vi "AuMT8852B EDR Carrier Frequency and Modulation Extended Results.vi"(5 "Stage":T1(ring), 8 "error in (no error)":errorcluster, 11 "VISA session":refnum<visa-resource-name>) -> (0 "error out":errorcluster, 2 "error code":i32, 3 "VISA session out":refnum<visa-resource-name>, 4 "Results":T2)   [LabVIEW 2017]
doc: "Anritsu MT8852B Bluetooth Tester\n\nReturns the results of the EDR Carrier Frequency Stability and Modulation test.\n\nINPUTS\nStage - results of the individual hopping stages of the test.\n\nOUTPUTS\nResults - measurements made during the test."
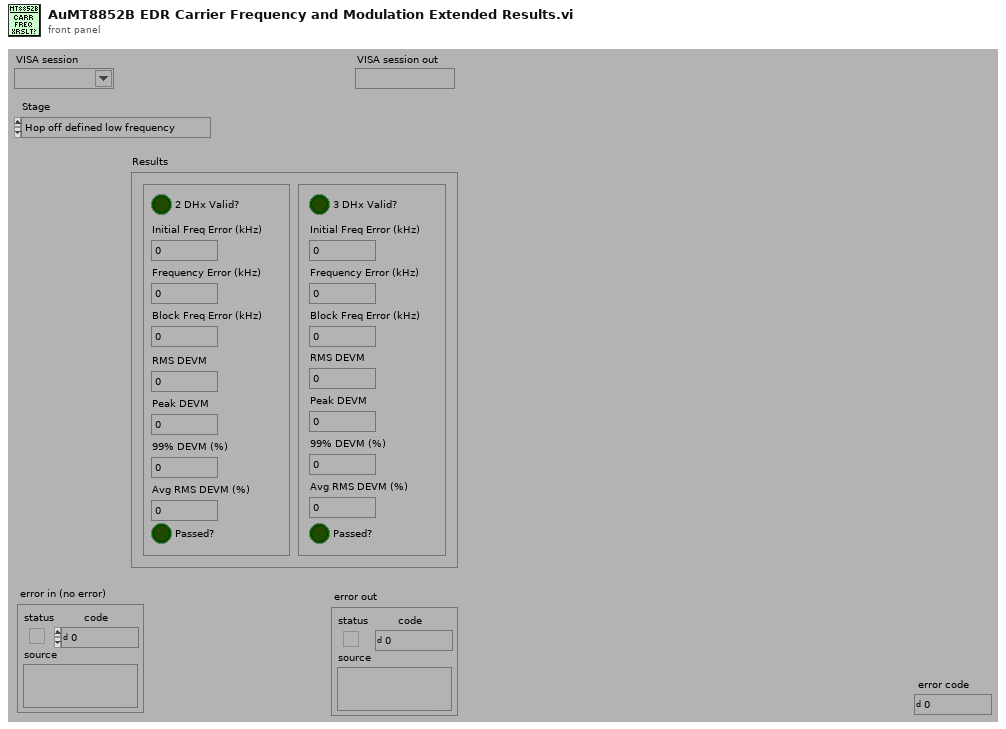
[diagram p1: front panel]
types:
  T1 = enum16{"Hop off defined low frequency", "Hop off defined medium frequency", "Hop off defined high frequency", "Hop on defined low frequency", "Hop on defined medium frequency", "Hop on defined high frequency", "Hop on all channels", "Hop on any channels"}
  T2 = cluster{"Passed?":bool, "RMS DEVM":sgl, "Peak DEVM":sgl, "99% DEVM (%)":sgl, "Avg RMS DEVM (%)":sgl, "Initial Freq Error (kHz)":sgl, "Frequency Error (kHz)":sgl, "Block Freq Error (kHz)":sgl, "2 DHx Valid?":bool, "Passed?":bool, "RMS DEVM":sgl, "Peak DEVM":sgl, "99% DEVM (%)":sgl, "Avg RMS DEVM (%)":sgl, "Initial Freq Error (kHz)":sgl, "Frequency Error (kHz)":sgl, "Block Freq Error (kHz)":sgl, "3 DHx Valid?":bool}
  T3 = enum16{"Simulate", "Range check", "Cache", "Query instrument status"}
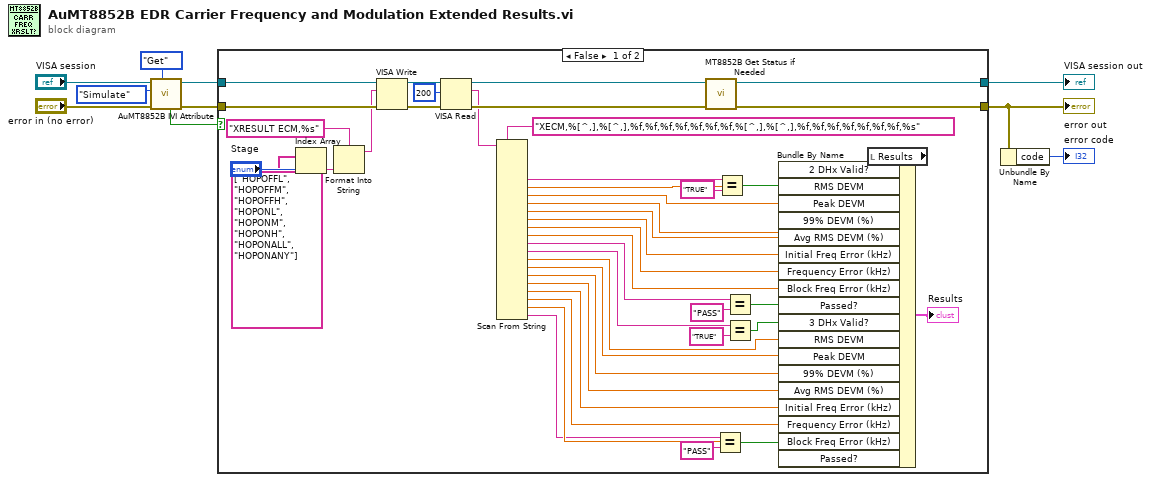
[diagram p0: block diagram]
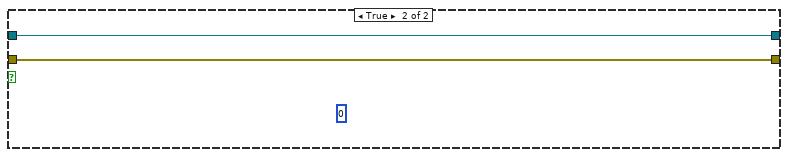
[diagram p2: hidden frame]
diagram:
  n1 = call <instrlib>:"AuMT8852B IVI Attribute.vi"("Set/Get (Set)"=enum16{"Set", "Get"}."Get", "error in (no error)"="error in (no error)", "Flag (Simulate)"=T3."Simulate", "VISA session"="VISA session") -> ("error out"=w7:errorcluster, "VISA session out"=w9:refnum<visa-resource-name>, "Value out"=w3:bool)  [unwired: 5 in]
  n2 = case shown="False" w3 {
    tunnel: [w48 w56] -> w10
    tunnel: [w47 w55] -> w1
    tunnel: w9 -> [w54 w56]
    tunnel: w7 -> [w53 w55]
    frame False {
      n3 = Index Array(array=string[] ["HOPOFFL", "HOPOFFM", "HOPOFFH", "HOPONL", "HOPONM", "HOPONH", "HOPONALL", "HOPONANY"], index="Stage") -> (element=w34:string)
      n4 = Format Into String(format string="XRESULT ECM,%s" ("write buffer (\"\")"), w34) -> (resulting string=w31:string)  [unwired: 2 in, 1 out]
      n5 = VISA Write(VISA resource name=w54, write buffer=w31, error in (no error)=w53) -> (VISA resource name out=w52:refnum<visa-resource-name>, error out=w51:errorcluster)  [unwired: 1 out]
      n6 = VISA Read(VISA resource name=w52, byte count=u32 200 ("byte count (0)"), error in (no error)=w51) -> (VISA resource name out=w46:refnum<visa-resource-name>, read buffer=w29:string, error out=w45:errorcluster)  [unwired: 1 out]
      n7 = Scan From String(format string="XECM,%[^,],%[^,],%f,%f,%f,%f,%f,%f,%f,%[^,],%[^,],%f,%f,%f,%f,%f,%f,%f,%s" ("Format String"), input string=w29) -> (output 2=w28:string, output 3=w27:dbl, output 4=w26:dbl, output 5=w25:dbl, output 6=w24:dbl, output 7=w23:dbl, output 8=w22:dbl, output 9=w21:dbl, output 10=w20:string, output 11=w19:string, output 12=w18:dbl, output 13=w17:dbl, output 14=w16:dbl, output 15=w15:dbl, output 16=w14:dbl, output 17=w13:dbl, output 18=w12:dbl, output 19=w11:string)  [unwired: 22 in, 3 out]
      n8 = call <instrlib>:"MT8852B Get Status if Needed.vi"("error in (no error)"=w45, "VISA session"=w46) -> ("error out"=w47:errorcluster, "VISA session out"=w48:refnum<visa-resource-name>)  [unwired: 8 in]
      n9 = Equal?(x=w11, y="PASS") -> (x = y?=w36:bool)
      n10 = Equal?(x=w28, y="TRUE") -> (x = y?=w42:bool)
      n11 = Equal?(x=w20, y="PASS") -> (x = y?=w39:bool)
      n12 = Equal?(x=w19, y="TRUE") -> (x = y?=w38:bool)
      n13 = local read "Results"() -> (w43:T2)
      n14 = Bundle By Name(cluster=w43, "2 DHx Valid?"=w42, "RMS DEVM"=w27, "Peak DEVM"=w26, "99% DEVM (%)"=w25, "Avg RMS DEVM (%)"=w24, "Initial Freq Error (kHz)"=w23, "Frequency Error (kHz)"=w22, "Block Freq Error (kHz)"=w21, "Passed?"=w39, "3 DHx Valid?"=w38, "RMS DEVM"=w18, "Peak DEVM"=w17, "99% DEVM (%)"=w16, "Avg RMS DEVM (%)"=w15, "Initial Freq Error (kHz)"=w14, "Frequency Error (kHz)"=w13, "Block Freq Error (kHz)"=w12, "Passed?"=w36) -> (→"Results":T2)
    }
    frame True {
      (unwired) u8 0
    }
  }
  "error out" <- w1
  "VISA session out" <- w10
  n15 = Unbundle By Name(w1) -> ("code"=→"error code":i32)
